vi "Create Task Wrapper.vi"(0 "Task map in":map{string, refnum<k21>}(c390), 5 "Message Data in":T3, 11 "error in (no error)":errorcluster) -> (4 "Task map out":map{string, refnum<k21>}(c390), 6 "Message Data out":T1, 15 "error out":errorcluster)   [LabVIEW 2021, in "NI DAQmx_wrapper.lvlib"]
uses:
  NI DAQmx_wrapper.lvlib
  NI DAQmx_server/RPC Messages/nidaqmx_grpc_CreateTaskRequest.ctl
  NI DAQmx_server/RPC Messages/nidevice_grpc_SessionInitializationBehavior.ctl
  NI DAQmx_server/RPC Messages/nidaqmx_grpc_CreateTaskResponse.ctl
  NI DAQmx_server/RPC Messages/nidevice_grpc_Session_session/nidevice_grpc_Session_session.lvclass
  NI DAQmx_server/RPC Messages/nidevice_grpc_Session.ctl
  TypeDefs/Create Task Inputs.ctl
  NI DAQmx_server/RPC Messages/nidevice_grpc_Session_session/nidevice_grpc_Session_session.lvclass/nidevice_grpc_Session_session.ctl
  <vilib>/Utility/error.llb/Error Cluster From Error Code.vi
  <vilib>/ErrorRing/Error Ring.xnode
  NI DAQmx_server/NI DAQmx_server.lvlib
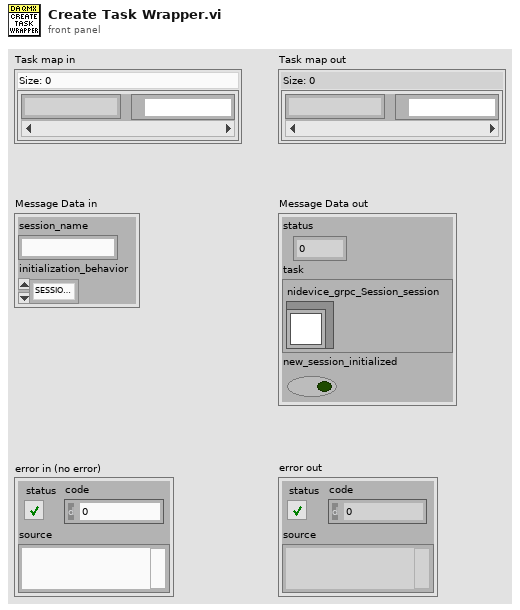
[diagram p1: front panel]
types:
  T1 = typedef "NI DAQmx_server.lvlib/nidaqmx_grpc_CreateTaskResponse.ctl" = cluster{"status":i32, "task":T2, "new_session_initialized":bool}
  T2 = typedef "NI DAQmx_server.lvlib/nidevice_grpc_Session.ctl" = cluster{"nidevice_grpc_Session_session":refnum<class "nidevice_grpc_Session_session.lvclass">}
  T3 = typedef "NI DAQmx_server.lvlib/nidaqmx_grpc_CreateTaskRequest.ctl" = cluster{"session_name":string, "initialization_behavior":T4}
  T4 = typedef "NI DAQmx_server.lvlib/nidevice_grpc_SessionInitializationBehavior.ctl" = enum32{"SESSION_INITIALIZATION_BEHAVIOR_UNSPECIFIED", "SESSION_INITIALIZATION_BEHAVIOR_INITIALIZE_NEW", "SESSION_INITIALIZATION_BEHAVIOR_ATTACH_TO_EXISTING"}
  T5 = typedef "NI DAQmx_wrapper.lvlib/Create Task Inputs.ctl" = cluster{"task to copy":refnum<k21>, "global virtual channels":refnum<k21>, "new task name":string, "auto cleanup":bool}
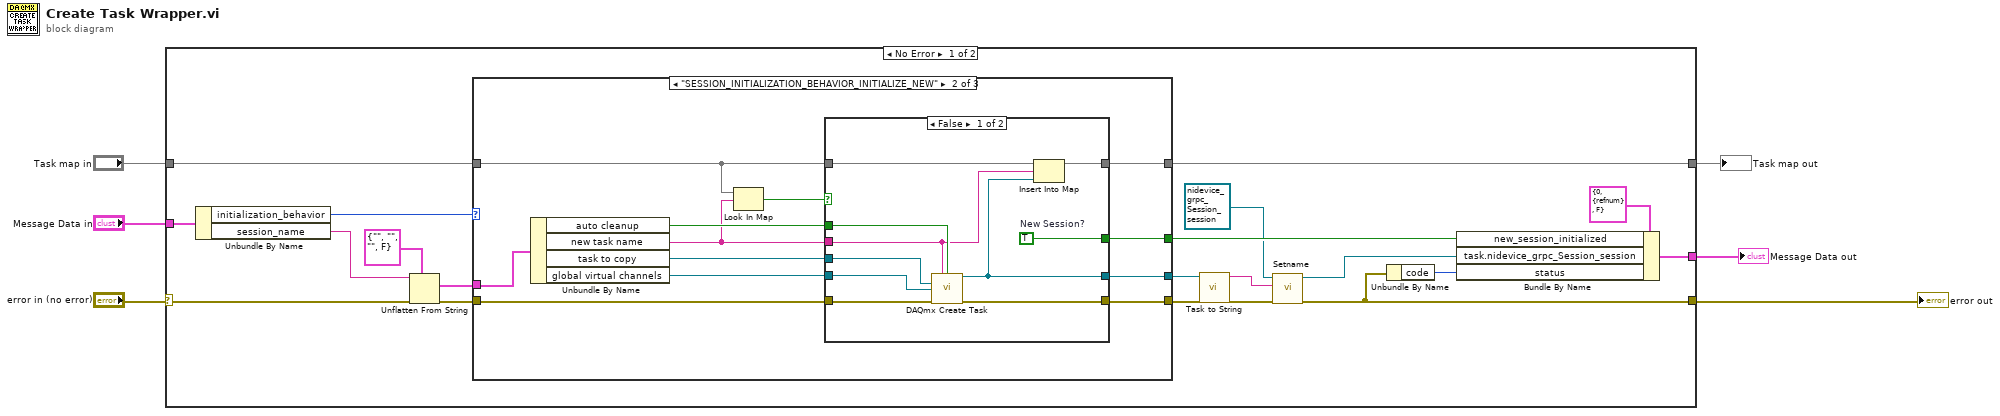
[diagram p0: block diagram]
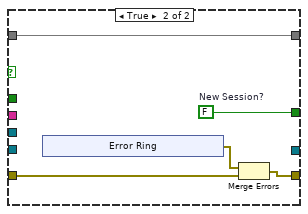
[diagram p3: hidden frame]
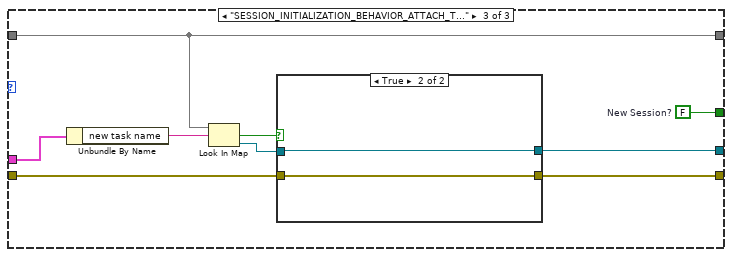
[diagram p4: hidden frame]
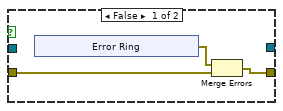
[diagram p5: hidden frame]
diagram:
  n1 = case shown="No Error" "error in (no error)" {
    selector: "error in (no error)" -> [w19 w80]
    tunnel: [w10 w80] -> w5
    tunnel: "Message Data in" -> [w25 _]
    tunnel: "Task map in" -> [w24 w79]
    tunnel: [w23 w79] -> w2
    tunnel: [w8 _] -> w1
    frame No Error {
      n2 = Unbundle By Name(w25) -> ("initialization_behavior"=w22:T4, "session_name"=w20:string)
      n3 = Unflatten From String(type=T5 {"task to copy"="", "global virtual channels"="", "new task name"="", "auto cleanup"=FALSE}, binary string=w20, error in (no error)=w19) -> (value=w17:T5, error out=w18:errorcluster)  [unwired: 2 in, 1 out]
      n4 = case shown="\"SESSION_INITIALIZATION_BEHAVIOR_INITIALIZE_NEW\"" w22 {
        tunnel: w24 -> [w27 w33 w67]
        tunnel: w18 -> [w26 w39 w63]
        tunnel: [w27 w34 w67] -> w23
        tunnel: w17 -> [_ w38 w68]
        tunnel: [w26 w30 w62] -> w13
        tunnel: [_ w29 w61] -> w15
        tunnel: [_ w28 w60] -> w14
        frame "SESSION_INITIALIZATION_BEHAVIOR_UNSPECIFIED", Default {
        }
        frame "SESSION_INITIALIZATION_BEHAVIOR_INITIALIZE_NEW" {
          n5 = Unbundle By Name(w38) -> ("auto cleanup"=w37:bool, "new task name"=w32:string, "task to copy"=w36:refnum<k21>, "global virtual channels"=w35:refnum<k21>)
          n6 = Look In Map(map=w33, key=w32) -> (key not found?=w31:bool)  [unwired: 1 in, 1 out]
          n7 = case shown="False" w31 {
            tunnel: w39 -> [w49 w53]
            tunnel: w37 -> [w48 _]
            tunnel: w36 -> [w47 _]
            tunnel: w35 -> [w46 _]
            tunnel: [w45 w50] -> w34
            tunnel: w33 -> [w44 w50]
            tunnel: w32 -> [w43 _]
            tunnel: [w42 w52] -> w30
            tunnel: [w41 w51] -> w29
            tunnel: [w40 _] -> w28
            frame False {
              w41 = TRUE  # New Session?
              n8 = call <vilib>:"DAQmx Create Task.vi"("new task name"=w43, "auto cleanup"=w48, "task to copy"=w47, "global virtual channels"=w46, "error in"=w49) -> ("task out"=w40:refnum<k21>, "error out"=w42:errorcluster)  [unwired: 9 in]
              n9 = Insert Into Map(map in=w44, key=w43, value=w40) -> (map out=w45:map{string, refnum<k21>})  [unwired: 2 out]
            }
            frame True {
              w51 = FALSE  # New Session?
              n10 = xnode "Error Ring"() -> ("error out"=w54:errorcluster)
              n11 = Merge Errors(w54, w53) -> (w52:errorcluster)
            }
          }
        }
        frame "SESSION_INITIALIZATION_BEHAVIOR_ATTACH_TO_EXISTING" {
          w61 = FALSE  # New Session?
          n12 = Unbundle By Name(w68) -> ("new task name"=w66:string)
          n13 = Look In Map(map=w67, key=w66) -> (key not found?=w65:bool, value=w64:refnum<k21>)  [unwired: 1 in]
          n14 = case shown="True" w65 {
            tunnel: w64 -> [_ w78]
            tunnel: w63 -> [w71 w77]
            tunnel: [_ w78] -> w60
            tunnel: [w69 w77] -> w62
            frame False {
              n15 = xnode "Error Ring"() -> ("error out"=w70:errorcluster)
              n16 = Merge Errors(w70, w71) -> (w69:errorcluster)
            }
            frame True {
            }
          }
        }
      }
      n17 = call "Task to String.vi"("Refnum in"=w14) -> ("String"=w12:string)  [unwired: 10 in]
      n18 = call "Setname.vi"("error in (no error)"=w13, "Set_Val"=w12, "OneOfTemplate in"=refnum<class "nidevice_grpc_Session_session.lvclass"> refnum) -> ("error out"=w10:errorcluster, "OneOfTemplate out"=w11:refnum<class "nidevice_grpc_Session_session.lvclass">)  [unwired: 7 in]
      n19 = Unbundle By Name(w10) -> ("code"=w9:i32)
      n20 = Bundle By Name(cluster=T1 {"status"=0, "task"={"nidevice_grpc_Session_session"=refnum}, "new_session_initialized"=FALSE} ("Message Data out"), "new_session_initialized"=w15, "task.nidevice_grpc_Session_session"=w11, "status"=w9) -> (w8:T1)
    }
    frame Error {
    }
  }
  "error out" <- w5
  "Task map out" <- w2
  "Message Data out" <- w1
